vi "RVC Drive in Circles.vi"() -> ()   [LabVIEW 2013]
uses:
  <vilib>/Simulation/Scripting/Companion Diagram/SimConfigNode/SimParams.ctl
  <vilib>/Simulation/Scripting/Companion Diagram/SimConfigNode/_simSolvers.ctl
  <vilib>/Simulation/Implementation/Shared/SIMSCR Execution Mode.ctl
  <vilib>/Simulation/Param Hierarchy/Typedefs/SIMPH Param Control Actions.ctl
  <vilib>/Simulation/Scripting/Editor Utilities/SIM subVI tag data.ctl
  <vilib>/Simulation/Scripting/Editor Utilities/SIM subVI execution type.ctl
  <vilib>/Simulation/Implementation/Shared/NILVSim_ParamChanged.vi
  <vilib>/Simulation/Implementation/Shared/NILVSIM_BeginStep.vi
  <vilib>/Simulation/Utility/Implementation/SIM Time.vi
  <vilib>/Simulation/SignalArithmetic/Implementation/NILVSim Gain.llb/SIM Gain (scalar).vi
  <vilib>/Simulation/Utility/Implementation/NILVSim Collector.llb/SIM Collector (vector).vi
  <vilib>/Simulation/Utility/Implementation/NILVSim Collector.llb/SIM Collector (scalar).vi
  <vilib>/Analysis/coordinate.llb/Wrap Angle.vi
  <vilib>/Analysis/coordinate.llb/Wrap Angle (scalar).vi
  <vilib>/Simulation/Implementation/Shared/SIM Fire Discrete SubVI.vi
  <vilib>/Simulation/Implementation/Shared/NILVSim_Manager.vi
  <vilib>/Simulation/Implementation/Shared/NILVSim_FinalizeModel.vi
  <vilib>/Simulation/Utility/Implementation/NILVSim Collector.llb/NILVSim Collector core (vector).vi
  <vilib>/Simulation/Utility/Implementation/NILVSim Collector.llb/NILVSim Collector core (scalar).vi
  <vilib>/Simulation/Implementation/Shared/SIM Fire Discrete SubVI (Core).vi
  <vilib>/Simulation/Implementation/Shared/SIM Unbundle Sim Info.vi
  <vilib>/Utility/error.llb/Clear Errors.vi
  <vilib>/Simulation/Implementation/Shared/NILVSim_GetModelError.vi
  <vilib>/Simulation/Implementation/Shared/SIM Bundle Sim Info.vi
  <vilib>/Simulation/Implementation/Shared/SIMSH Read Queue.vi
  <vilib>/Simulation/Implementation/Shared/NILVSim_Initialize.vi
  <vilib>/Simulation/Utility/Implementation/NILVSim Get Time and IsAcceptedStep.vi
  subVIs/2D Animate Rotating Wheel.vi
  subVIs/2D Animation.vi
  <vilib>/Simulation/Scripting/Companion Diagram/SimConfigNode/SimDog.xnode
  SIM Bicycle.vi
  <vilib>/Simulation/Model Libraries/PID/SIM PID (Parallel).vi
  <vilib>/Simulation/Model Libraries/PID/SIM PID.vi
  <vilib>/Simulation/Implementation/XNodeFramework/SimXNode/SimX.xnode
  <vilib>/Analysis/NI_AAL_Angle.lvlib
  <vilib>/Simulation/Implementation/Shared/NI_SIM_Implementation.lvlib
panel:
  out "XY Graph 3":cluster{"Time":dbl[], "Signal":dbl[]}(graph)
  out "XY Graph 2":cluster{"Signal":dbl[], "Signal":dbl[]}(graph)
  out "Position":cluster{"x":dbl, "y":dbl, "theta":dbl}
  out "Angle (deg)":dbl format="%.2f"
  out "Steering Angle":picture
  out "Goal":dbl[](array[numeric])
  out "Map Floor":picture
  out "velocity":dbl(knob)=1.0 scale=0.0..2.0
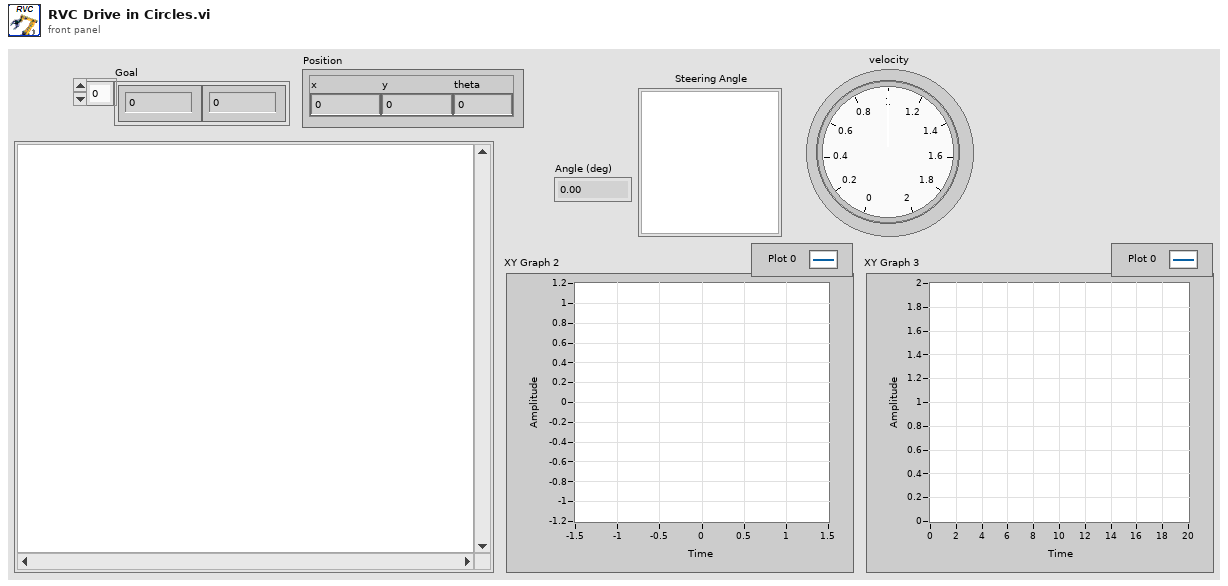
[diagram p1: front panel]
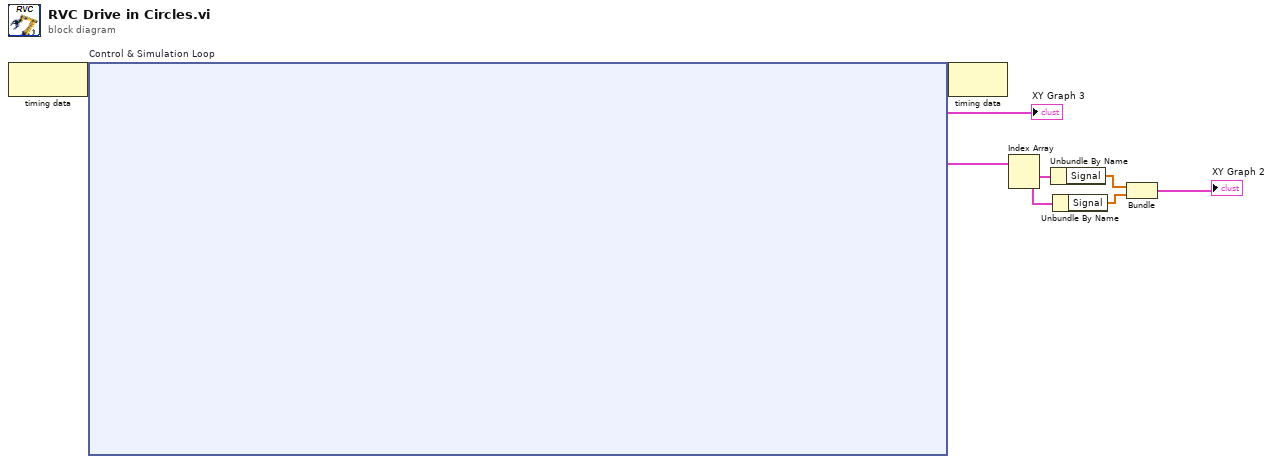
[diagram p0: block diagram]
diagram:
  n1 = node-c288() -> (w8:variant)  [unwired: 1 in]
  n2 = node-c254 "Control & Simulation Loop"(w8) -> (w7:variant, w6:cluster{"Time":dbl[], "Signal":dbl[]}[], →"XY Graph 3":cluster{"Time":dbl[], "Signal":dbl[]})
  n3 = node-c288(w7) -> ()  [unwired: 1 out]
  n4 = Index Array(array=w6) -> (element #1=w5:cluster{"Time":dbl[], "Signal":dbl[]}, element #2=w4:cluster{"Time":dbl[], "Signal":dbl[]})  [unwired: 2 in]
  n5 = Unbundle By Name(w5) -> ("Signal"=w3:dbl[])
  n6 = Unbundle By Name(w4) -> ("Signal"=w2:dbl[])
  n7 = Bundle("Signal"=w3, "Signal"=w2) -> (→"XY Graph 2":cluster{"Signal":dbl[], "Signal":dbl[]})  [unwired: 1 in]
